vi "Actor Core.vi"(8 "error in":errorcluster, 11 "Auto UI in":refnum<class "Auto UI.lvclass">) -> (0 "error out":errorcluster, 3 "Actor out":refnum<class "Actor.lvclass">)   [LabVIEW 2023, in "GUI.lvlib" / "Auto UI.lvlib" / "Auto UI.lvclass"]
doc: "(<B>Filename</B>: Actor Framework.lvlib:Actor.lvclass:Actor Core.vi)\n\nReceives messages to the actor, reacts to them, and initiates any error handling that may shut the actor down.\n\nDescendant classes may override this VI to append parallel tasks for the actor to complete while it handles messages. Overrides use the Call Parent Class Method node."
uses:
  Auto UI.lvclass
  C:/Program Files/National Instruments/LabVIEW 2023/vi.lib/ActorFramework/Actor/Actor.lvclass
  <vilib>/ActorFramework/Actor/Actor.lvclass
  Typdefs/Auto GUI/Remaining Duration.ctl
  Typdefs/Auto GUI/Test Info.ctl
  Typdefs/Auto GUI/Cycles and Mode.ctl
  Typdefs/Auto GUI/Software Description.ctl
  Typdefs/Auto GUI/Temperature Display.ctl
  Typdefs/Auto GUI/Additional Data.ctl
  Typdefs/Auto GUI/Duration.ctl
  Auto UI.lvclass/Auto UI.ctl
  <vilib>/ActorFramework/Actor/Actor.lvclass/Actor.ctl
  <vilib>/ActorFramework/Message Enqueuer/Message Enqueuer.lvclass/Message Enqueuer.ctl
  Reused Code/Subpanels Actor/subpanels/subpanel Messages/Insert Msg/Insert Msg.lvclass/Insert Msg.ctl
  Main/Main Messages/MenuBar Visable Msg/MenuBar Visable Msg.lvclass/MenuBar Visable Msg.ctl
  <vilib>/ActorFramework/Message Enqueuer/Init from Existing Queue.vi
  <vilib>/ActorFramework/Message Enqueuer/Enqueue.vi
  Reused Code/Subpanels Actor/subpanels/subpanel Messages/Insert Msg/Insert Msg.lvclass
  C:/Program Files/National Instruments/LabVIEW 2023/vi.lib/ActorFramework/Message/Message.lvclass
  Reused Code/Subpanels Actor/subpanels/subpanel (abstract) Messages/Initialize SP Msg/Initialize SP Msg.lvclass
  Auto UI Messages/TS Station Global Update UI Msg/TS Station Global Update UI Msg.lvclass
  Main/Main Messages/MenuBar Visable Msg/MenuBar Visable Msg.lvclass
  <vilib>/ActorFramework/Message Priority Queue/Priority Enqueue.vi
  <vilib>/ActorFramework/Message Enqueuer/Message Enqueuer.lvclass
  Reused Code/Subpanels Actor/subpanels/subpanel/subpanel (abstract).lvclass
  D:/eDCU LTT/VT LTT Project/Source Code/GUI/Reused Code/Subpanels Actor/subpanels/subpanel/subpanel (abstract).lvclass
  D:/eDCU LTT/VT LTT Project/Source Code/GUI/Actor/Auto UI/Auto UI/Auto UI.lvclass
  GUI.lvlib
panel:
  out "Duration":T1={"Completed Duration"="ABCD", "Remaining Duration"="ABCD"}
  out "Test Prograss(%)":dbl(slide)=1.0 scale=0.0..100.0
  out "Completed Percentage":dbl format="%#.1f%"
  out "Estimated Date:":string
  out "Completed Duration":T2 {"Day" format="%02d"; "Min" format="%02d"; "Hours" format="%02d"}
  out "Additional Data":T3
  out "Temperature Display":T4
  out "Software Version":T5
  out "Cycles and Mode":T6
  out "Test Info":T7={"Project Name"="ABCD", "Product Name"="ABCD", "Product Varient"="ABCD", "Test Name"="ABCD", "Test Start Time"="ABCD", "Estimated Date"="ABCD"}
  out "Remaining Duration":T2 {"Day" format="%02d"; "Min" format="%02d"; "Hours" format="%02d"}
  out "Error LED":bool=TRUE
  out "Status LED":bool=TRUE
  out "Status":string="abcd"
  in  "Open Seq File":bool caption="Blank"
  in  "Stop Test":bool caption="Blank"
  in  "Pause":bool caption="Blank"
  in  "Start":bool=TRUE caption="Blank"
  in  "Stop":bool
  in  "Terminate All Button":refnum<k7>(container)
  in  "Exit Button":refnum<k7>(container)
  in  "Login/Logout Button":refnum<k7>(container)
  in  "Close Executions Button":refnum<k7>(container)
  in  "Break/Resume Button":refnum<k7>(container)
  in  "Terminate/Restart Button":refnum<k7>(container)
  in  "Run Selected Sequence Button":refnum<k7>(container)
  in  "Entry Point 2 Button":refnum<k7>(container)
  in  "Entry Point 1 Button":refnum<k7>(container)
  in  "Report Viewer":refnum<k7>(container)
  in  "Close Sequence File Button":refnum<k7>(container)
  in  "Open Sequence File Button":refnum<k7>(container)
  in  "Executions ComboBox":refnum<k7>(container) caption="Executions:"
  in  "Sequences ComboBox":refnum<k7>(container) caption="Sequences:"
  in  "Execution View":refnum<k7>(container)
  in  "Sequence Files ComboBox":refnum<k7>(container) caption="Sequence Files:"
  in  "ExecutionView Manager":refnum<k7>(container)
  in  "SequenceFileView Manager":refnum<k7>(container)
  # "Test Panel"
  # "Test Info"
  # "Execution View"
  # "Software Info"
  # "Temperature Info"
  # "Error Info"
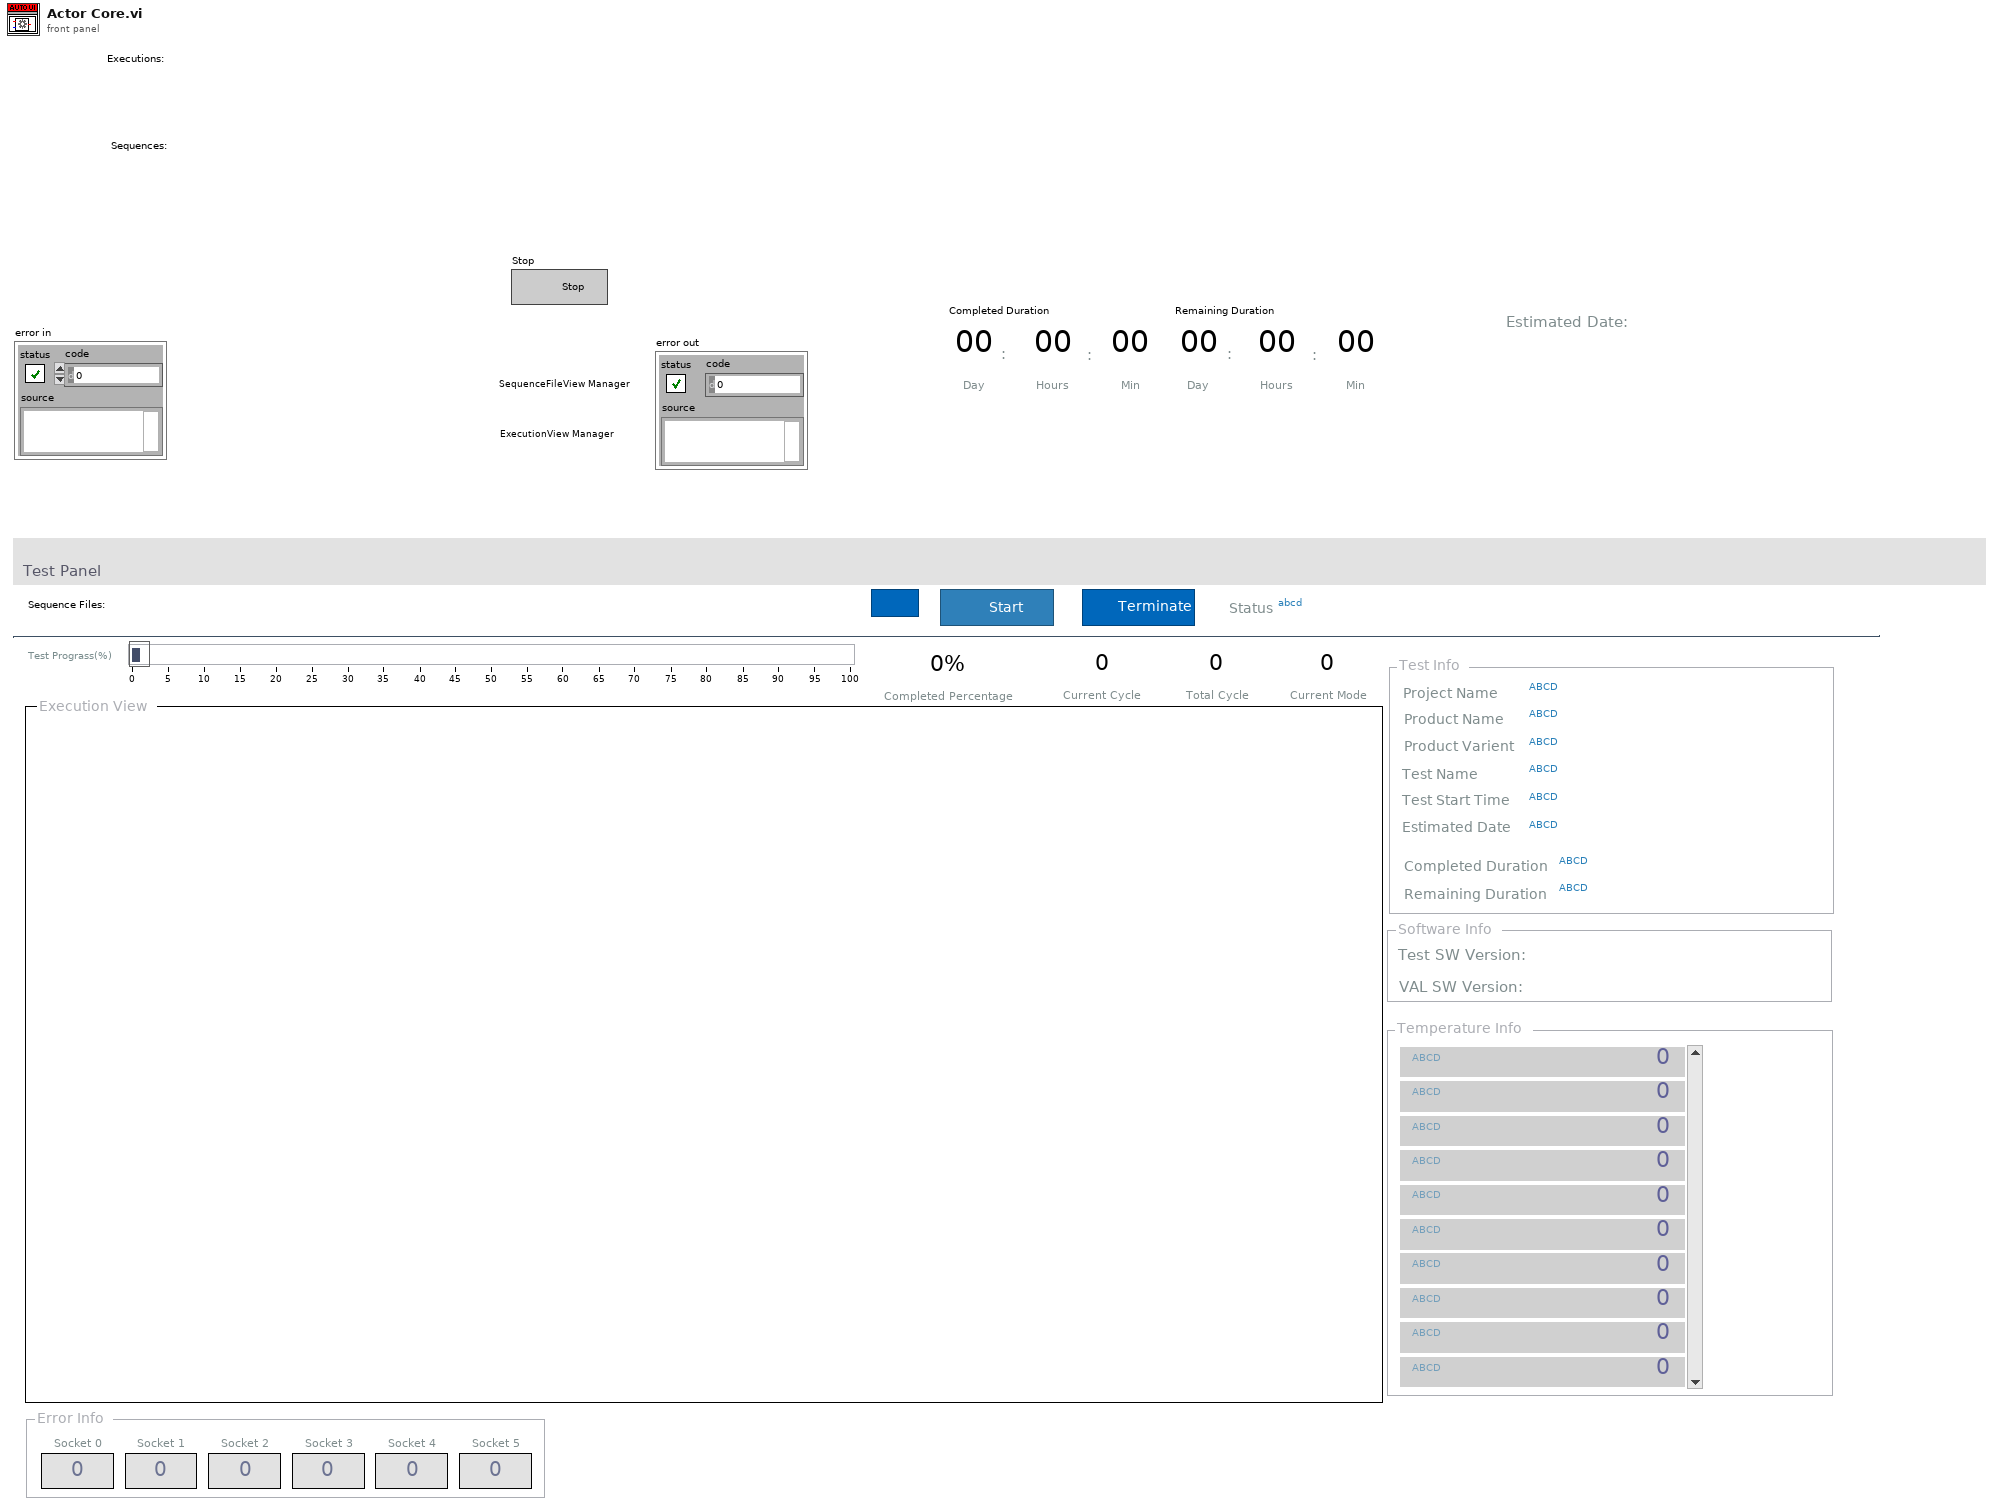
[diagram p1: front panel]
types:
  T1 = typedef "GUI.lvlib/Duration.ctl" = cluster{"Completed Duration":string, "Remaining Duration":string}
  T2 = typedef "GUI.lvlib/Remaining Duration.ctl" = cluster{"Hours":u8, "Min":u8, "Day":u8}
  T3 = typedef "GUI.lvlib/Additional Data.ctl" = cluster{"Socket 0":u32, "Socket 1":u32, "Socket 2":u32, "Socket 3":u32, "Socket 4":u32, "Socket 5":u32}
  T4 = typedef "GUI.lvlib/Temperature Display.ctl" = cluster{"Temperature Name":string, "Temperature":i32}[]
  T5 = typedef "GUI.lvlib/Software Description.ctl" = cluster{"Test SW Version:":string, "VAL SW Version:":string}
  T6 = typedef "GUI.lvlib/Cycles and Mode.ctl" = cluster{"Current Cycle":u32, "Total Cycle":u32, "Current Mode":u32}
  T7 = typedef "GUI.lvlib/Test Info.ctl" = cluster{"Project Name":string, "Product Name":string, "Product Varient":string, "Test Name":string, "Test Start Time":string, "Estimated Date":string}
  T8 = enum8{"Enabled", "Disabled", "Disabled and Grayed Out"}
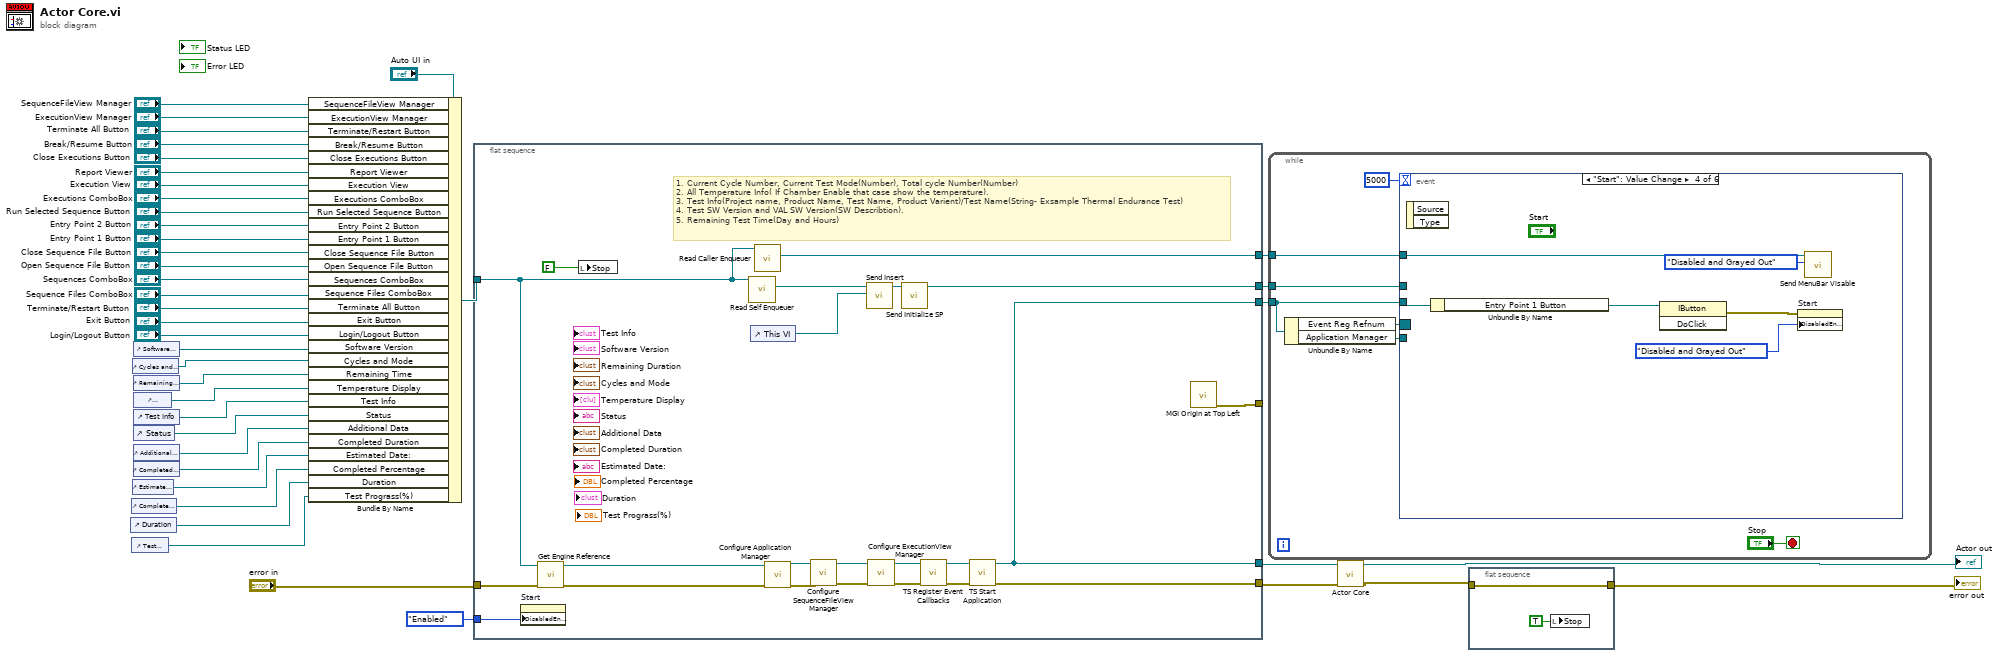
[diagram p0: block diagram]
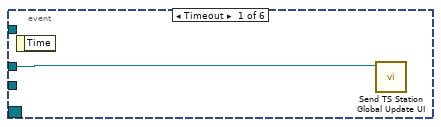
[diagram p2: hidden frame]
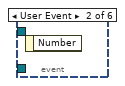
[diagram p3: hidden frame]
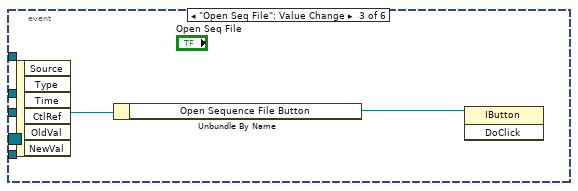
[diagram p4: hidden frame]
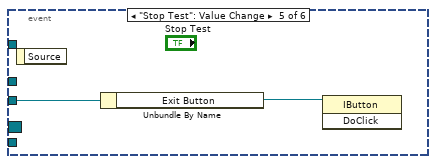
[diagram p5: hidden frame]
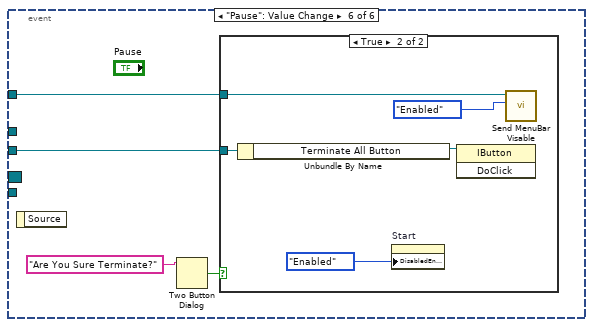
[diagram p6: hidden frame]
diagram:
  n1 = control-ref of="Duration"() -> (w3:refnum<vi>)
  n2 = control-ref of="Completed Percentage"() -> (w4:refnum<vi>)
  n3 = control-ref of="Test Prograss(%)"() -> (w2:refnum<vi>)
  n4 = control-ref of="Cycles and Mode"() -> (w13:refnum<vi>)
  n5 = control-ref of="Estimated Date:"() -> (w5:refnum<vi>)
  n6 = control-ref of="Software Version"() -> (w14:refnum<vi>)
  n7 = control-ref of="Remaining Duration"() -> (w12:refnum<vi>)
  n8 = control-ref of="Temperature Display"() -> (w11:refnum<vi>)
  n9 = control-ref of="Test Info"() -> (w10:refnum<vi>)
  n10 = control-ref of="Status"() -> (w9:refnum<vi>)
  n11 = control-ref of="Additional Data"() -> (w7:refnum<vi>)
  n12 = control-ref of="Completed Duration"() -> (w6:refnum<vi>)
  n13 = Bundle By Name(cluster="Auto UI in", "SequenceFileView Manager"="SequenceFileView Manager", "ExecutionView Manager"="ExecutionView Manager", "Terminate/Restart Button"="Terminate All Button", "Break/Resume Button"="Break/Resume Button", "Close Executions Button"="Close Executions Button", "Report Viewer"="Report Viewer", "Execution View"="Execution View", "Executions ComboBox"="Executions ComboBox", "Run Selected Sequence Button"="Run Selected Sequence Button", "Entry Point 2 Button"="Entry Point 2 Button", "Entry Point 1 Button"="Entry Point 1 Button", "Close Sequence File Button"="Close Sequence File Button", "Open Sequence File Button"="Open Sequence File Button", "Sequences ComboBox"="Sequences ComboBox", "Sequence Files ComboBox"="Sequence Files ComboBox", "Terminate All Button"="Terminate/Restart Button", "Exit Button"="Exit Button", "Login/Logout Button"="Login/Logout Button", "Software Version"=w14, "Cycles and Mode"=w13, "Remaining Time"=w12, "Temperature Display"=w11, "Test Info"=w10, "Status"=w9, "Additional Data"=w7, "Completed Duration"=w6, "Estimated Date:"=w5, "Completed Percentage"=w4, "Duration"=w3, "Test Prograss(%)"=w2) -> (w21:refnum<class "Auto UI.lvclass">)
  n14 = flat-sequence {
    tunnel: "error in" -> [w64]
    tunnel: [w48] -> w15
    tunnel: [w54] -> w22
    tunnel: w21 -> [w46]
    tunnel: [w49] -> w20
    tunnel: [w48] -> w17
    tunnel: [w45] -> w8
    tunnel: [w44] -> _
    tunnel: T8."Enabled" ("Disabled") -> [w43]
    frame #0 {
      # "1. Current Cycle Number, Current Test Mode(Number), Total cycle Number(Number)\n2. All Temperature Info( If Chamber Enable that case show the temperature).\n3. Test Info(Project name, Product Name, Test Name, Product Varient)/Test Name(String- Exsample Thermal Endurance Test)\n4. Test SW Version and VAL SW Version(SW Describtion).\n5. Remaining Test Time(Day and Hours)"
      n15 = property on="Start" class="Bool (strict)"("DisabledEnum"=w43) -> ()  [unwired: 2 in, 2 out]
      n16 = call "Get Engine Reference.vi"("error in (no error)"=w64, "Auto UI in"=w46) -> ("error out"=w47:errorcluster, "Auto UI out"=w55:refnum<class "Auto UI.lvclass">)  [unwired: 8 in]
      n17 = local write "Stop"(FALSE ("Stop Button")) -> ()
      n18 = call <vilib>:"Read Self Enqueuer.vi"("Actor"=w46) -> ("Self Enqueuer"=w53:refnum<class "Message Enqueuer.lvclass">)  [unwired: 10 in]
      n19 = control-ref of="This VI"() -> (w52:refnum<vi>)
      n20 = call <vilib>:"Read Caller Enqueuer.vi"("Actor"=w46) -> ("Caller Enqueuer"=w45:refnum<class "Message Enqueuer.lvclass">)  [unwired: 10 in]
      n21 = call "Configure Application Manager.vi"("error in (no error)"=w47, "Auto UI in"=w55) -> ("error out"=w62:errorcluster, "Auto UI out"=w63:refnum<class "Auto UI.lvclass">)  [unwired: 8 in]
      n22 = call "Configure SequenceFileView Manager.vi"("error in (no error)"=w62, "Auto UI in"=w63) -> ("error out"=w61:errorcluster, "Auto UI out"=w60:refnum<class "Auto UI.lvclass">)  [unwired: 8 in]
      n23 = call "Send Insert.vi"("VI Ref"=w52, "Message Enqueuer"=w53) -> ("Message Enqueuer out"=w51:refnum<class "Message Enqueuer.lvclass">)  [unwired: 8 in, 1 out]
      n24 = call "Configure ExecutionView Manager.vi"("error in (no error)"=w61, "Auto UI in"=w60) -> ("error out"=w59:errorcluster, "Auto UI out"=w58:refnum<class "Auto UI.lvclass">)  [unwired: 8 in]
      n25 = call "Send Initialize SP.vi"("Message Enqueuer"=w51) -> ("Message Enqueuer out"=w49:refnum<class "Message Enqueuer.lvclass">)  [unwired: 9 in, 1 out]
      n26 = call "TS Register Event Callbacks.vi"("error in (no error)"=w59, "Auto UI in"=w58) -> ("error out"=w57:errorcluster, "Auto UI out"=w56:refnum<class "Auto UI.lvclass">)  [unwired: 8 in]
      n27 = call "TS Start Application.vi"("error in (no error)"=w57, "Auto UI in"=w56) -> ("error out"=w54:errorcluster, "Auto UI out"=w48:refnum<class "Auto UI.lvclass">)  [unwired: 8 in]
      n28 = call <userlib>:"MGI Origin at Top Left.vi"() -> ("Error Out"=w44:errorcluster)  [unwired: 9 in, 1 out]
    }
  }
  n29 = while {
    tunnel: w20 -> [w69]
    tunnel: w17 -> [w68]
    tunnel: w8 -> [w65]
    stop <- "Stop" stop-if-true
    n30 = Unbundle By Name(w68) -> ("Event Reg Refnum"=w67:refnum<event-registration>, "Application Manager"=w66:refnum<k7>)
    n31 = event shown="[3] \"Start\": Value Change" {
      selector: w67 -> [_ _ _ _ _ _]
      dyn-events: _ -> [_ _ _ _ _ _]
      timeout: 5000 -> [_ _ _ _ _ _]
      tunnel: w69 -> [w72 _ _ _ _ _]
      tunnel: w68 -> [_ _ w74 w80 w82 w86]
      tunnel: w66 -> [_ _ _ _ _ _]
      tunnel: w65 -> [_ _ _ w78 _ w85]
      event Timeout {
        n32 = event-data() -> ()  [unwired: 1 in, 1 out]
        n33 = call "Send TS Station Global Update UI.vi"("Message Enqueuer"=w72) -> ()  [unwired: 9 in, 2 out]
      }
      event User Event {
        n34 = event-data() -> ()  [unwired: 1 in, 1 out]
      }
      event "Open Seq File": Value Change {
        n35 = event-data() -> ()  [unwired: 1 in, 6 out]
        n36 = Unbundle By Name(w74) -> ("Open Sequence File Button"=w73:refnum<k7>)
        n37 = invoke class="IButton" method="DoClick"(reference=w73) -> ()  [unwired: 2 in, 3 out]
      }
      event "Start": Value Change {
        n38 = event-data() -> ()  [unwired: 1 in, 2 out]
        n39 = Unbundle By Name(w80) -> ("Entry Point 1 Button"=w79:refnum<k7>)
        n40 = invoke class="IButton" method="DoClick"(reference=w79) -> (error out=w76:errorcluster)  [unwired: 2 in, 2 out]
        n41 = property on="Start" class="Bool (strict)"(error in=w76, "DisabledEnum"=T8."Disabled and Grayed Out" ("Disabled")) -> ()  [unwired: 1 in, 2 out]
        n42 = call "Send MenuBar Visable.vi"("Disabled"=T8."Disabled and Grayed Out", "Message Enqueuer"=w78) -> ()  [unwired: 8 in, 2 out]
      }
      event "Stop Test": Value Change {
        n43 = event-data() -> ()  [unwired: 1 in, 1 out]
        n44 = Unbundle By Name(w82) -> ("Exit Button"=w81:refnum<k7>)
        n45 = invoke class="IButton" method="DoClick"(reference=w81) -> ()  [unwired: 2 in, 3 out]
      }
      event "Pause": Value Change {
        n46 = event-data() -> ()  [unwired: 1 in, 1 out]
        n47 = Two Button Dialog(message="Are You Sure Terminate?") -> (T button?=w83:bool)  [unwired: 2 in]
        n48 = case shown="True" w83 {
          tunnel: w86 -> [_ w91]
          tunnel: w85 -> [_ w89]
          frame False {
          }
          frame True {
            n49 = Unbundle By Name(w91) -> ("Terminate All Button"=w90:refnum<k7>)
            n50 = property on="Start" class="Bool (strict)"("DisabledEnum"=T8."Enabled" ("Disabled")) -> ()  [unwired: 2 in, 2 out]
            n51 = invoke class="IButton" method="DoClick"(reference=w90) -> ()  [unwired: 2 in, 3 out]
            n52 = call "Send MenuBar Visable.vi"("Disabled"=T8."Enabled", "Message Enqueuer"=w89) -> ()  [unwired: 8 in, 2 out]
          }
        }
      }
    }
  }
  n53 = call-parent "Actor Core.vi"("error in"=w22, "Actor in"=w15) -> ("error out"=w19:errorcluster, "Actor out"=→"Actor out":refnum<class "Actor.lvclass">)  [unwired: 8 in]
  n54 = flat-sequence {
    tunnel: w19 -> [w92]
    tunnel: [w92] -> w18
    frame #0 {
      n55 = local write "Stop"(TRUE ("Stop")) -> ()
    }
  }
  "error out" <- w18
